vi "EventLog.Confirm(error).vi"(8 "error in":errorcluster, 9 "current time":timestamp, 10 "ErrData":T1) -> (0 "error out":errorcluster)   [LabVIEW 2013]
uses:
  EventLog.EventLevel.ctl
  Translator/Translator.Message.ctl
  EventLog.EventGui.ctl
  EventLog.Buffer.Action.ctl
  EventLog.Event.ctl
  Global/ApplicationGlobal.vi
  User/User.Global.vi
  EventLog.EventSource.ctl
  CitTemplate/citTemplate.errData.ctl
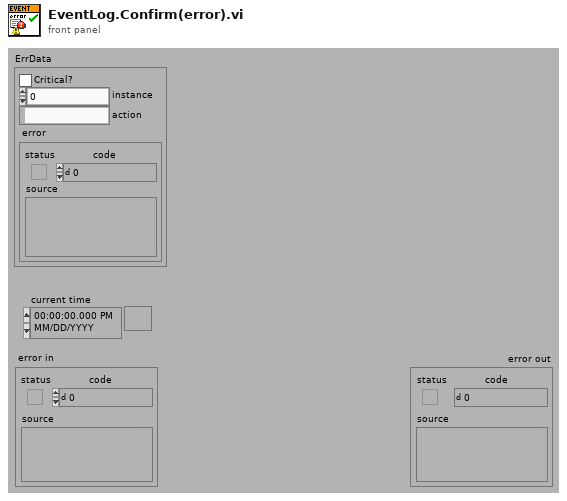
[diagram p1: front panel]
types:
  T1 = typedef "citTemplate.errData.ctl" = cluster{"Critical?":bool, "instance":i32, "action":string, "error":errorcluster}
  T2 = typedef "EventLog.Event.ctl" = cluster{"ts":dbl, "lev":T3, "usr":i32, "source":T4, "msg":T5, "arg":variant[]}
  T3 = typedef "EventLog.EventLevel.ctl" = enum8{"Debug", "Info", "Warning", "Error", "Critical"}
  T4 = typedef "EventLog.EventSource.ctl" = enum16{"App", "Gui", "DB", "Seq", "File", "DIO", "AI", "AO", "IFM", "CPX"}
  T5 = typedef "Translator.Message.ctl" = enum16{"-", "Log out", "Log in", "Shutdown", "Cancel", "Start", "Error %d >> %s", "Error %d >> %s >> %s", "Error %d confirmed", "Error %d cleared", "Starting %s", "Quitting %s", "User %s level %s added", "User %s level %s deleted", "User %s level %s changed to %s", "Initializing...", "Quitting...", "Loading...", "Do you want to continue?", "Calibration", "Log out?", "System", "All", "IDLE", "Translating...%s", "Not found", "Alarm %s", "Restart is required to translate the application! Do you want to restart the PC?", "Restart cancelled. Be aware that some controls may not be fully translated until you restart the application.", "New version available!", "The software is up-to-date", "PC software will be updated after rebooting the PC. Do you want to reboot now?", "RT software will be updated. Make sure that no process is running. Do you want to reboot RT now?", "Updating RT firmware. Please wait...", "Update failed: %s", "Rebooting...", "Rebooting RT. Please wait...", "RT updated to version %s", "Timeout error during update. Check if RT is working", "Run", "Skip", "Abort", "Please wait...", "Put reference number...", "Seq: Folder '%s' is missing", "Seq: File '%s' is missing", "Seq: File '%s' is broken", "Seq: File '%s' is running", "Seq: Test steps are missing", "DB: Incorrect settings", "DB: Initializing...", "DB: ERR%d >> %s", "DB: OK", "Daq: DI #%d and #%d have share the same resource", "Daq: DO #%d and #%d have share the same resource", "Daq: DIO Incorrect settings", "Daq: AI Incorrect settings", "Daq: DIO Initializing...", "Daq: AI Initializing...", "Daq: DIO ERR%d >> %s", "Daq: AI ERR%d >> %s", "Daq: DIO OK", "Daq: AI OK"}
  T6 = typedef "EventLog.Buffer.Action.ctl" = enum16{"init", "re-init", "clear", "set translator", "add", "get"}
  T7 = typedef "EventLog.EventGui.ctl" = cluster{"ts":dbl, "lev":T3, "usr":i32, "source":T4, "msg":T5, "arg":variant[], "msg_str":string}
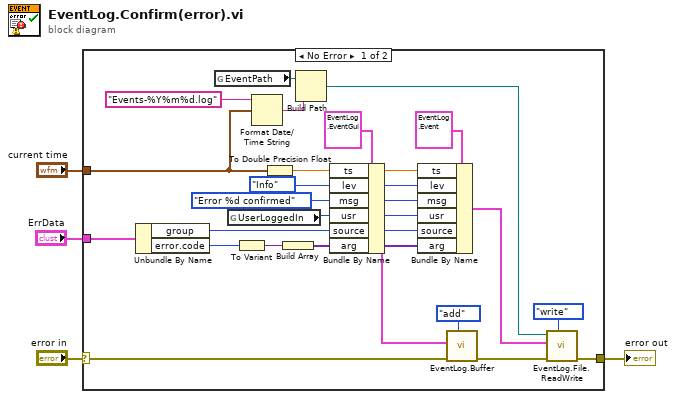
[diagram p0: block diagram]
diagram:
  n1 = case shown="No Error" "error in" {
    selector: "error in" -> [w10 w28]
    tunnel: [w23 w28] -> w4
    tunnel: "ErrData" -> [w13 _]
    tunnel: "current time" -> [w6 _]
    frame No Error {
      w7 = EventLog.EventLevel."Info" ("lev")
      w20 = Translator.Message."Error %d confirmed" ("msg")
      n2 = Unbundle By Name(w13) -> ("group"=w8:T4, "error.code"=w12:i32)
      n3 = global read "ApplicationGlobal.vi" "EventPath"() -> (w17:path)
      n4 = global read "User.Global.vi" "UserLoggedIn"() -> (w14:i32)
      n5 = To Variant(anything=w12) -> (Variant=w11:variant)
      n6 = Format Date/Time String(time format string (%c)="Events-%Y%m%d.log", seconds (now)=w6) -> (date/time string=w16:string)  [unwired: 1 in]
      n7 = To Double Precision Float(number=w6) -> (double precision float=w21:dbl)
      n8 = Build Array(w11) -> (w5:variant[])
      n9 = Build Path(base path=w17, name or relative path=w16) -> (appended path=w15:path)
      n10 = Bundle By Name(cluster=T7 {"ts"=0.0, "lev"=enum."Debug", "usr"=0, "source"=enum."App", "msg"=enum."Log out", "arg"=[], "msg_str"=""} ("Event in"), "ts"=w21, "lev"=w7, "msg"=w20, "usr"=w14, "source"=w8, "arg"=w5) -> (w9:T7)
      n11 = Bundle By Name(cluster=T2 {"ts"=0.0, "lev"=enum."Debug", "usr"=0, "source"=enum."App", "msg"=enum."Log out", "arg"=[]} ("event in"), "ts"=w21, "lev"=w7, "msg"=w20, "usr"=w14, "source"=w8, "arg"=w5) -> (w19:T2)
      n12 = call "EventLog.Buffer.vi"("action (get)"=EventLog.Buffer.Action."add" ("action (read)"), "error in"=w10, "Event in"=w9) -> ("error out"=w24:errorcluster)  [unwired: 6 in, 2 out]
      n13 = call "EventLog.File.ReadWrite.vi"("action (read)"=enum16{"read", "write"}."write", "error in"=w24, "event in"=w19, "file"=w15) -> ("error out"=w23:errorcluster)  [unwired: 3 in, 4 out]
    }
    frame Error {
    }
  }
  "error out" <- w4
